vi "Update beam locations.vi"(8 "error in (no error)":errorcluster, 9 "New location":dbl, 10 "Beam on cup":T1(radio)=enum."Bottom Cup on Beam", 11 "Lifter_motor in":refnum<class "Lifter_motor.lvclass">) -> (0 "error out":errorcluster, 3 "Lifter_motor out":refnum<class "Lifter_motor.lvclass">)   [LabVIEW 2019, in "Lifter_motor.lvclass"]
uses:
  Lifter_motor.lvclass
  Lifter_motor.lvclass/Lifter_motor.ctl
panel:
  out "output array":dbl[](array[numeric])
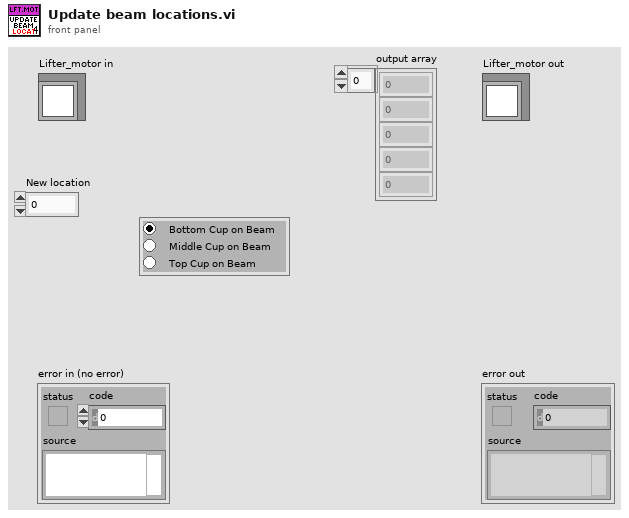
[diagram p1: front panel]
types:
  T1 = enum32{"No Selection", "Bottom Cup on Beam", "Middle Cup on Beam", "Top Cup on Beam"}
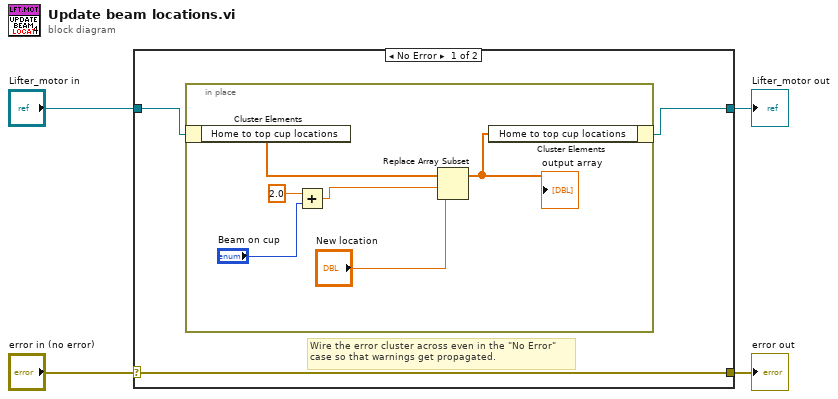
[diagram p0: block diagram]
diagram:
  n1 = case shown="No Error" "error in (no error)" {
    selector: "error in (no error)" -> [w7 w15]
    tunnel: [w7 w15] -> w3
    tunnel: [w5 w14] -> w1
    tunnel: "Lifter_motor in" -> [w6 w14]
    frame No Error {
      # "Wire the error cluster across even in the \"No Error\"\ncase so that warnings get propagated."
      n2 = in-place {
        n3 = in-place-cluster #1(w6) -> ("Home to top cup locations"=w9:dbl[])
        n4 = Add(x=2.0, y="Beam on cup") -> (x+y=w13:dbl)
        n5 = Replace Array Subset(array=w9, new element="New location", index=w13) -> (w8:dbl[])
        "output array" <- w8
        n6 = in-place-cluster #1("Home to top cup locations"=w8) -> (w5:refnum<class "Lifter_motor.lvclass">)
      }
    }
    frame Error {
    }
  }
  "error out" <- w3
  "Lifter_motor out" <- w1
